vi "ROI group-Set number of sel groups ind.vi"(8 "error in (no error)":errorcluster) -> (0 "error out":errorcluster)   [LabVIEW 2013]
uses:
  Global variables/gl_Functional Imaging-Global variables.vi
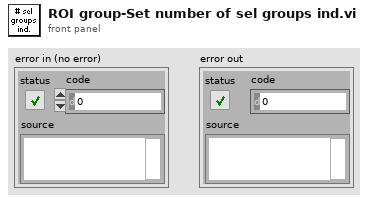
[diagram p1: front panel]
types:
  T1 = typedef "Functional Imging UI Refs.ctl" = cluster{"Menu ref":refnum<k9>, "Image control":refnum<vi>, "VI ref":refnum<vi>, "XGrapher":refnum<vi>, "Smoothing":refnum<vi>, "POI Averaging":refnum<vi>, "Normalize":refnum<vi>, "POI data points in each trial":refnum<vi>, "Channel":refnum<vi>, "Experiment data folder path":refnum<vi>, "[ROI vis]":refnum<vi>, "[Groups] visbl":T2, "Group Name":refnum<vi>, "POI index":refnum<vi>, "Trial No.":refnum<vi>, "Intensity Zoom":refnum<vi>, "Trial Cursor Enabled":refnum<vi>, "Number of Trials (ind 1)":refnum<vi>, "Number of Trials (ind 2)":refnum<vi>, "MiniScans Available":refnum<vi>, "POI Available":refnum<vi>, "Defer graph updates":refnum<vi>, "Waveform selector":refnum<vi>, "#of selected POI":refnum<vi>, "#of selected MiniScans":refnum<vi>, "#of selected groups":refnum<vi>, "Max Z-Projection":refnum<vi>, "Z-Plane Selector":refnum<vi>, "Index of miniscan point to visualise":refnum<vi>, "ROI vis. mode":refnum<vi>, "Total # of points":refnum<vi>, "Index of group clicked on":refnum<vi>, "Pane 1":refnum<vi>, "Pane 2":refnum<vi>, "Pane 3":refnum<vi>, "Pane 4":refnum<vi>, "Pane 5":refnum<vi>, "Pane 6":refnum<vi>, "Deselect all ROI":refnum<vi>, "Deselect all groups":refnum<vi>}
  T2 = typedef "Groups array referecne.ctl" = refnum<vi>
  T3 = typedef "Group sel cluster.ctl" = cluster{"Group number":string, "Group Name":string, "Visibility":bool, "Highlight":bool}
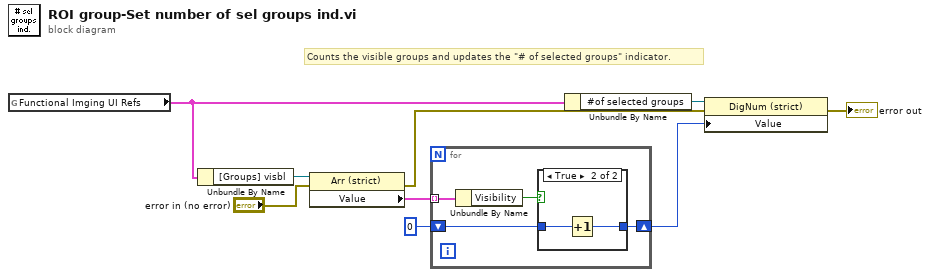
[diagram p0: block diagram]
diagram:
  # "Counts the visible groups and updates the \"# of selected groups\" indicator."
  n1 = global read "gl_Functional Imaging-Global variables.vi" "Functional Imging UI Refs"() -> (w6:T1)
  n2 = Unbundle By Name(w6) -> ("[Groups] visbl"=w7:T2)
  n3 = property on="Property Node" class="Arr (strict)"(reference=w7, error in="error in (no error)") -> (error out=w1:errorcluster, "Value"=w4:T3[])  [unwired: 1 out]
  n4 = for {
    tunnel: w4 -> [w13] mode=indexing
    shift-right: [w10] -> w2
    shift-left: 0 -> [w11]
    n5 = Unbundle By Name(w13) -> ("Visibility"=w12:bool)
    n6 = case shown="True" w12 {
      tunnel: w11 -> [w14 w16]
      tunnel: [w14 w15] -> w10
      frame False {
      }
      frame True {
        n7 = Increment(x=w16) -> (x+1=w15:i32)
      }
    }
  }
  n8 = Unbundle By Name(w6) -> ("#of selected groups"=w8:refnum<vi>)
  n9 = property on="Property Node" class="DigNum (strict)"(reference=w8, error in=w1, "Value"=w2) -> (error out=→"error out":errorcluster)  [unwired: 1 out]
